vi "Get Alarm Screencap Variables.vi"(8 "error in (no error)":errorcluster, 11 "LabVIEW Web Service Request":refnum<class "Web Request.lvclass">) -> (0 "error out":errorcluster, 3 "LabVIEW Web Service Request out":refnum<class "Web Request.lvclass">)   [LabVIEW 2018]
doc: "This VI sets all of the ESP variables for a single contact so it can be output from an ESP script."
uses:
  <vilib>/wsapi/Web Request.lvclass
  CAEN globals.vi
  <vilib>/wsapi/class/subVIs/Set String ESP Variable.vi
panel:
  out "result string":string
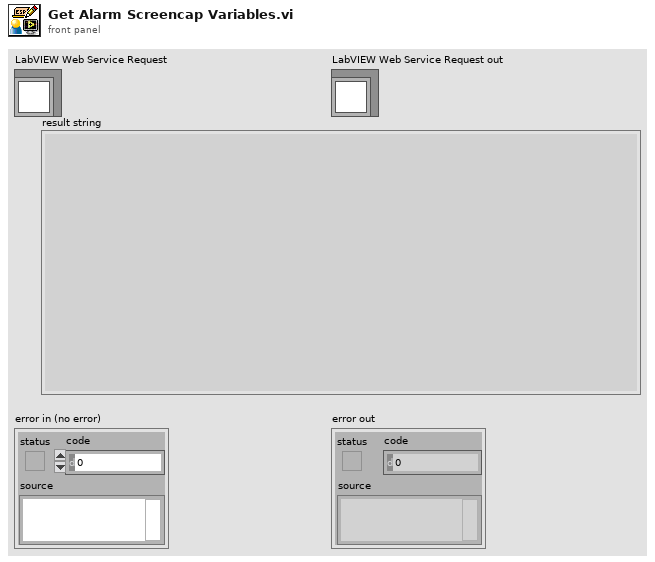
[diagram p1: front panel]
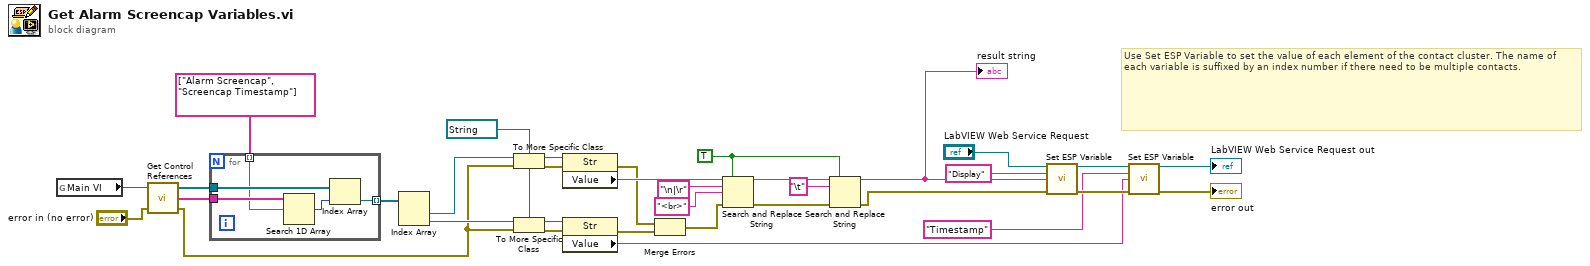
[diagram p0: block diagram]
diagram:
  w10 = refnum<vi> refnum ("reference out")
  w25 = TRUE ("replace all? (F)")
  # "Use Set ESP Variable to set the value of each element of the contact cluster. The name of each variable is suffixed by an index number if there need to be multiple contacts."
  n1 = global read "CAEN globals.vi" "Main VI"() -> (w23:refnum<vi>)
  n2 = call "Get Control References.vi"("error in"="error in (no error)", "This vi"=w23) -> ("error out"=w11:errorcluster, "Control Names"=w22:string[], "Controls[]"=w21:refnum<vi>[])  [unwired: 1 in]
  n3 = for {
    tunnel: w22 -> [w39]
    tunnel: w21 -> [w37]
    tunnel: [w36] -> w16 mode=indexing
    tunnel: string[] ["Alarm Screencap", "Screencap Timestamp"] ("Control Names") -> [w35] mode=indexing
    n4 = Search 1D Array(1D array=w39, element=w35) -> (index of element=w38:i32)  [unwired: 1 in]
    n5 = Index Array(array=w37, index=w38) -> (element=w36:refnum<vi>)
  }
  n6 = Index Array(array=w16) -> (element #1=w15:refnum<vi>, element #2=w12:refnum<vi>)  [unwired: 2 in]
  n7 = To More Specific Class(target class=w10, reference=w15, error in=w11) -> (specific class reference=w18:refnum<vi>, error out=w17:errorcluster)
  n8 = To More Specific Class(target class=w10, reference=w12, error in=w11) -> (specific class reference=w13:refnum<vi>, error out=w14:errorcluster)
  n9 = property class="Str"(reference=w18, error in=w17) -> (error out=w9:errorcluster, "Value"=w30:string)  [unwired: 1 out]
  n10 = property class="Str"(reference=w13, error in=w14) -> (error out=w7:errorcluster, "Value"=w2:string)  [unwired: 1 out]
  n11 = Merge Errors(w9, w7) -> (w8:errorcluster)
  n12 = Search and Replace String(replace all?=w25, input string=w30, search string="\n|\r", replace string="<br>" ("search string"), error in=w8) -> (result string=w27:string, error out=w29:errorcluster)  [unwired: 3 in, 2 out]
  n13 = Search and Replace String(replace all?=w25, input string=w27, search string="\t", error in=w29) -> (result string=w26:string, error out=w28:errorcluster)  [unwired: 4 in, 2 out]
  "result string" <- w26
  n14 = call-poly <vilib>:"Set ESP Variable.vi"("LabVIEW Web Service Request"="LabVIEW Web Service Request", "key"="Display" ("format string"), "value"=w26, "error in (no error)"=w28) -> ("LabVIEW Web Service Request out"=w4:refnum<class "Web Request.lvclass">, "error out"=w6:errorcluster)  [unwired: 10 in]
  n15 = call-poly <vilib>:"Set ESP Variable.vi"("LabVIEW Web Service Request"=w4, "key"="Timestamp" ("format string"), "value"=w2, "error in (no error)"=w6) -> ("LabVIEW Web Service Request out"=→"LabVIEW Web Service Request out":refnum<class "Web Request.lvclass">, "error out"=→"error out":errorcluster)  [unwired: 10 in]
